vi "InternalStructPos.vi"() -> ()   [LabVIEW 2015]
uses:
  GlobalPath.vi
  GlobalData.vi
  GlobalVi.vi
panel:
  in  "ptfe 9":bool caption="Position the 2 cooling bars"
  in  "Done?":bool
  in  "ptfe 6":bool caption="Connect the mass ground jumpers among the 6 external frames"
  in  "ptfe 5":bool caption="Screw the 20 mass grounds to the frames (internal+external)"
  in  "ptfe 4":bool caption="Position the 5 honeycomb sheets"
  in  "ptfe 3":bool caption="Position the 4 internal frames"
  in  "ptfe 2":bool caption="Position the 6 external frames using 12 PTFE pins"
  # "Internal Structure Positioning"
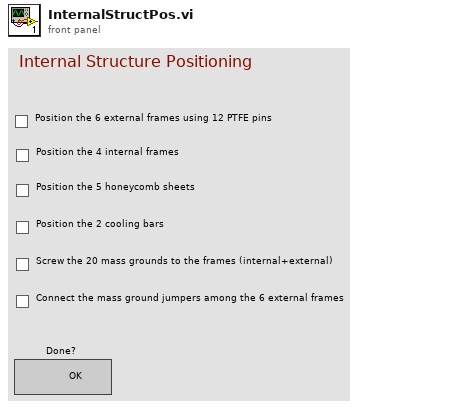
[diagram p1: front panel]
types:
  T1 = enum16{"open", "replace", "create", "open or create", "replace or create", "replace or create with confirmation"}
  T2 = enum32{"Bad", "Idle", "Run top level", "Running"}
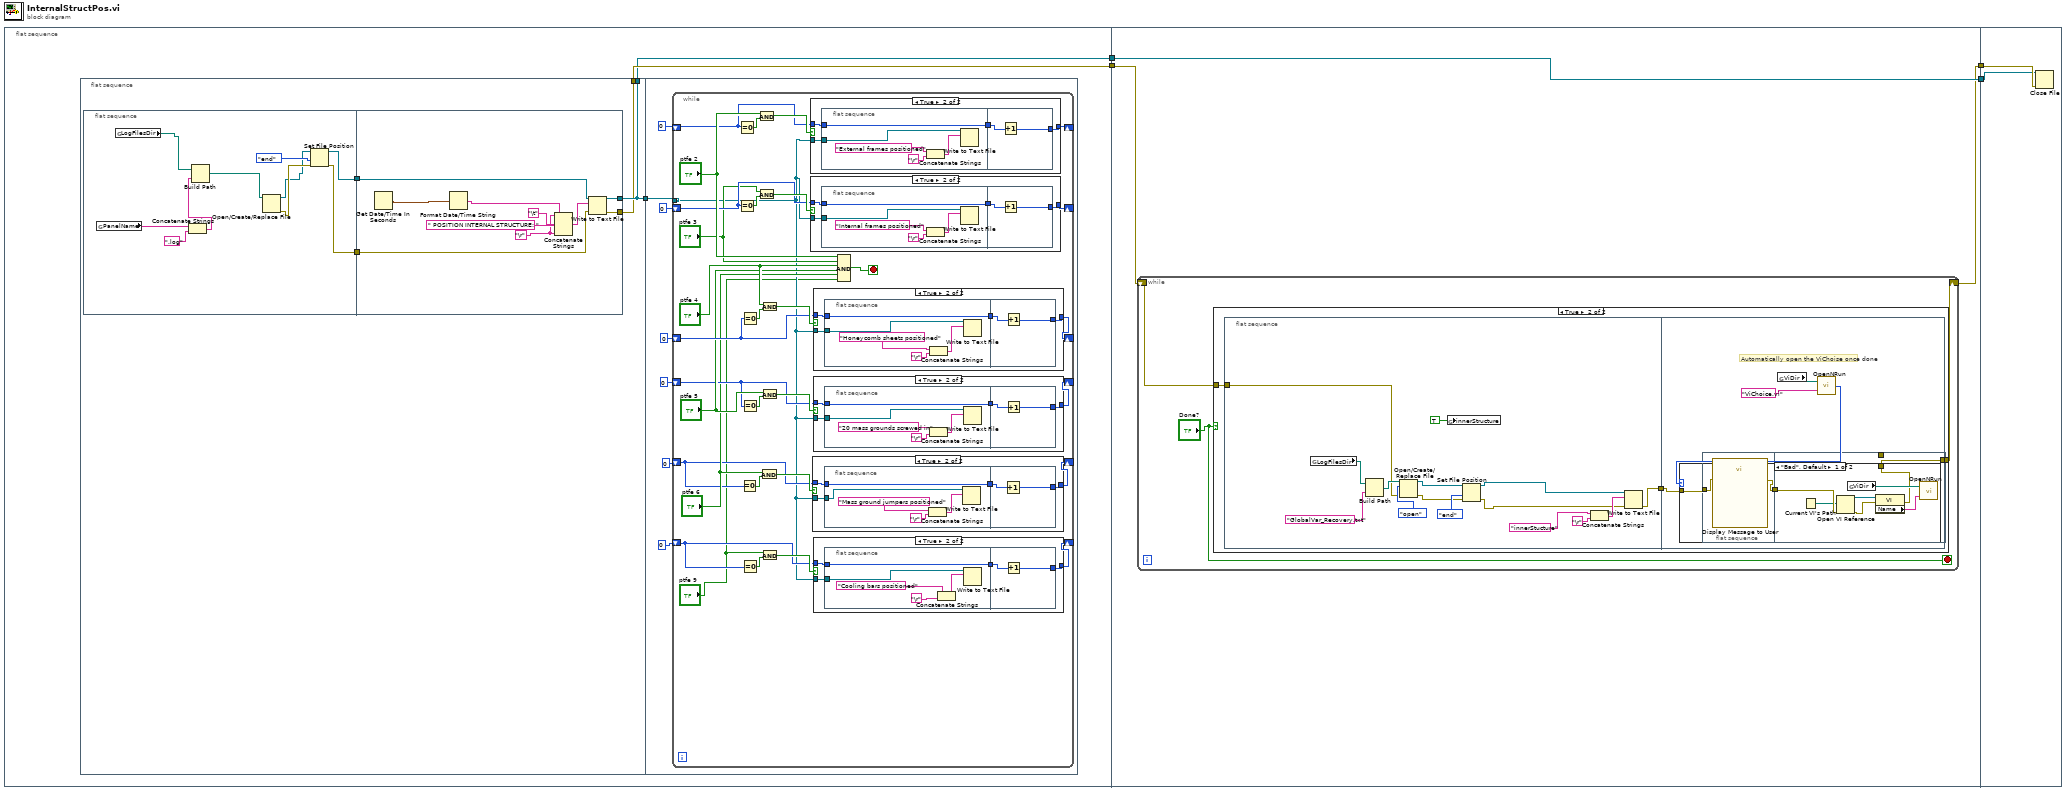
[diagram p0: block diagram]
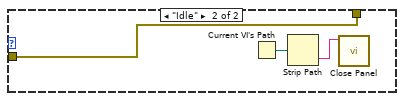
[diagram p9: hidden frame]
diagram:
  n1 = flat-sequence {
    tunnel: [w6] -> w3
    tunnel: [w5] -> w2
    tunnel: [w144] -> w4
    tunnel: w3 -> [w143]
    tunnel: w2 -> [w145]
    tunnel: [w145] -> w1
    tunnel: w4 -> [w189]
    tunnel: w1 -> [w188]
    frame #0 {
      n2 = flat-sequence {
        tunnel: [w10] -> w7
        tunnel: [w10] -> w5
        tunnel: [w9] -> w6
        tunnel: w7 -> [w38]
        frame #0 {
          n3 = flat-sequence {
            tunnel: [w13] -> w11
            tunnel: [w15] -> w8
            tunnel: w11 -> [w27]
            tunnel: [w26] -> w10
            tunnel: [w25] -> w9
            tunnel: w8 -> [w24]
            frame #0 {
              n4 = global read "GlobalData.vi" "PanelName"() -> (w20:string)
              n5 = global read "GlobalPath.vi" "LogFilesDir"() -> (w12:path)
              n6 = Concatenate Strings(w20, ".log") -> (w19:string)
              n7 = Build Path(base path=w12, name or relative path=w19) -> (appended path=w18:path)
              n8 = Open/Create/Replace File(file path (use dialog)=w18) -> (refnum out=w14:refnum<file>, error out=w16:errorcluster)  [unwired: 5 in, 1 out]
              n9 = Set File Position(refnum=w14, from (0:start)=enum16{"start", "end", "current"}."end", error in=w16) -> (refnum out=w13:refnum<file>, error out=w15:errorcluster)  [unwired: 1 in]
            }
            frame #1 {
              w22 = "\r"
              n10 = Get Date/Time In Seconds() -> (seconds since 1Jan1904=w23:timestamp)
              n11 = Format Date/Time String(seconds (now)=w23) -> (date/time string=w29:string)  [unwired: 2 in]
              n12 = Concatenate Strings(w22, w29, "\t", " POSITION INTERNAL STRUCTURE: ", w22) -> (w28:string)
              n13 = Write to Text File(file (use dialog)=w27, text=w28, error in=w24) -> (refnum out=w26:refnum<file>, error out=w25:errorcluster)  [unwired: 1 in, 1 out]
            }
          }
        }
        frame #1 {
          n14 = while {
            tunnel: w38 -> [w40]
            shift-right: [w65] -> _
            shift-left: 0 -> [w66]
            shift-right: [w61] -> _
            shift-left: 0 -> [w62]
            shift-right: [w55] -> _
            shift-left: 0 -> [w57]
            shift-right: [w50] -> _
            shift-left: 0 -> [w51]
            shift-right: [w45] -> _
            shift-left: 0 -> [w46]
            shift-right: [w41] -> _
            shift-left: 0 -> [w42]
            stop <- w70 stop-if-true
            n15 = Equal To 0?(x=w66) -> (x = 0?=w69:bool)
            n16 = Equal To 0?(x=w62) -> (x = 0?=w64:bool)
            n17 = Equal To 0?(x=w46) -> (x = 0?=w49:bool)
            n18 = Equal To 0?(x=w57) -> (x = 0?=w59:bool)
            n19 = Equal To 0?(x=w51) -> (x = 0?=w54:bool)
            n20 = Equal To 0?(x=w42) -> (x = 0?=w44:bool)
            n21 = And(x="ptfe 2", y=w69) -> (x .and. y?=w68:bool)
            n22 = And(x="ptfe 3", y=w64) -> (x .and. y?=w63:bool)
            n23 = And(x="ptfe 6", y=w49) -> (x .and. y?=w48:bool)
            n24 = And(x="ptfe 4", y=w59) -> (x .and. y?=w58:bool)
            n25 = And(x="ptfe 5", y=w54) -> (x .and. y?=w53:bool)
            n26 = And(x="ptfe 9", y=w44) -> (x .and. y?=w43:bool)
            n27 = case shown="True" w68 {
              tunnel: w40 -> [_ w135]
              tunnel: w66 -> [w131 w133]
              tunnel: [w131 w132] -> w65
              frame False {
              }
              frame True {
                n28 = flat-sequence {
                  tunnel: w135 -> [w138]
                  tunnel: [w137] -> w134
                  tunnel: w133 -> [w137]
                  tunnel: w134 -> [w142]
                  tunnel: [w141] -> w132
                  frame #0 {
                    n29 = Concatenate Strings("External frames positioned", "\r") -> (w140:string)
                    n30 = Write to Text File(file (use dialog)=w138, text=w140) -> ()  [unwired: 2 in, 3 out]
                  }
                  frame #1 {
                    n31 = Increment(x=w142) -> (x+1=w141:i32)
                  }
                }
              }
            }
            n32 = case shown="True" w63 {
              tunnel: w40 -> [_ w123]
              tunnel: w62 -> [w119 w121]
              tunnel: [w119 w120] -> w61
              frame False {
              }
              frame True {
                n33 = flat-sequence {
                  tunnel: w123 -> [w126]
                  tunnel: [w125] -> w122
                  tunnel: w121 -> [w125]
                  tunnel: w122 -> [w130]
                  tunnel: [w129] -> w120
                  frame #0 {
                    n34 = Concatenate Strings("Internal frames positioned", "\r") -> (w128:string)
                    n35 = Write to Text File(file (use dialog)=w126, text=w128) -> ()  [unwired: 2 in, 3 out]
                  }
                  frame #1 {
                    n36 = Increment(x=w130) -> (x+1=w129:i32)
                  }
                }
              }
            }
            n37 = case shown="True" w48 {
              tunnel: w40 -> [_ w87]
              tunnel: w46 -> [w83 w85]
              tunnel: [w83 w84] -> w45
              frame False {
              }
              frame True {
                n38 = flat-sequence {
                  tunnel: w87 -> [w90]
                  tunnel: [w89] -> w86
                  tunnel: w85 -> [w89]
                  tunnel: w86 -> [w94]
                  tunnel: [w93] -> w84
                  frame #0 {
                    n39 = Concatenate Strings("Mass ground jumpers positioned", "\r") -> (w92:string)
                    n40 = Write to Text File(file (use dialog)=w90, text=w92) -> ()  [unwired: 2 in, 3 out]
                  }
                  frame #1 {
                    n41 = Increment(x=w94) -> (x+1=w93:i32)
                  }
                }
              }
            }
            n42 = case shown="True" w58 {
              tunnel: w40 -> [_ w111]
              tunnel: w57 -> [w107 w109]
              tunnel: [w107 w108] -> w55
              frame False {
              }
              frame True {
                n43 = flat-sequence {
                  tunnel: w111 -> [w114]
                  tunnel: [w113] -> w110
                  tunnel: w109 -> [w113]
                  tunnel: w110 -> [w118]
                  tunnel: [w117] -> w108
                  frame #0 {
                    n44 = Concatenate Strings("Honeycomb sheets positioned", "\r") -> (w116:string)
                    n45 = Write to Text File(file (use dialog)=w114, text=w116) -> ()  [unwired: 2 in, 3 out]
                  }
                  frame #1 {
                    n46 = Increment(x=w118) -> (x+1=w117:i32)
                  }
                }
              }
            }
            n47 = case shown="True" w53 {
              tunnel: w40 -> [_ w99]
              tunnel: w51 -> [w95 w97]
              tunnel: [w95 w96] -> w50
              frame False {
              }
              frame True {
                n48 = flat-sequence {
                  tunnel: w99 -> [w102]
                  tunnel: [w101] -> w98
                  tunnel: w97 -> [w101]
                  tunnel: w98 -> [w106]
                  tunnel: [w105] -> w96
                  frame #0 {
                    n49 = Concatenate Strings("20 mass grounds screwed in", "\r") -> (w104:string)
                    n50 = Write to Text File(file (use dialog)=w102, text=w104) -> ()  [unwired: 2 in, 3 out]
                  }
                  frame #1 {
                    n51 = Increment(x=w106) -> (x+1=w105:i32)
                  }
                }
              }
            }
            n52 = case shown="True" w43 {
              tunnel: w40 -> [_ w75]
              tunnel: w42 -> [w71 w73]
              tunnel: [w71 w72] -> w41
              frame False {
              }
              frame True {
                n53 = flat-sequence {
                  tunnel: w75 -> [w78]
                  tunnel: [w77] -> w74
                  tunnel: w73 -> [w77]
                  tunnel: w74 -> [w82]
                  tunnel: [w81] -> w72
                  frame #0 {
                    n54 = Concatenate Strings("Cooling bars positioned", "\r") -> (w80:string)
                    n55 = Write to Text File(file (use dialog)=w78, text=w80) -> ()  [unwired: 2 in, 3 out]
                  }
                  frame #1 {
                    n56 = Increment(x=w82) -> (x+1=w81:i32)
                  }
                }
              }
            }
            n57 = Compound Arithmetic op=AND("ptfe 2", "ptfe 3", "ptfe 4", "ptfe 5", "ptfe 6", "ptfe 9") -> (w70:bool)
          }
        }
      }
    }
    frame #1 {
      n58 = while {
        shift-right: [w148] -> w144
        shift-left: w143 -> [w147]
        stop <- "Done?" stop-if-true
        n59 = case shown="True" "Done?" {
          tunnel: [w149 w152] -> w148
          tunnel: w147 -> [w149 w151]
          frame False {
          }
          frame True {
            n60 = flat-sequence {
              tunnel: w151 -> [w156]
              tunnel: [w155] -> w150
              tunnel: [w169] -> w152
              tunnel: w150 -> [w168]
              frame #0 {
                n61 = global read "GlobalPath.vi" "LogFilesDir"() -> (w153:path)
                n62 = Build Path(base path=w153, name or relative path="GlobalVar_Recovery.txt") -> (appended path=w165:path)
                n63 = Open/Create/Replace File(file path (use dialog)=w165, error in=w156, operation (0:open)=T1."open") -> (refnum out=w161:refnum<file>, error out=w162:errorcluster)  [unwired: 3 in, 1 out]
                n64 = global write "GlobalVi.vi" "innerStructure"(TRUE) -> ()
                n65 = Set File Position(refnum=w161, from (0:start)=enum16{"start", "end", "current"}."end", error in=w162) -> (refnum out=w158:refnum<file>, error out=w157:errorcluster)  [unwired: 1 in]
                n66 = Concatenate Strings("innerStucture", "\r") -> (w160:string)
                n67 = Write to Text File(file (use dialog)=w158, text=w160, error in=w157) -> (error out=w155:errorcluster)  [unwired: 1 in, 2 out]
              }
              frame #1 {
                # "Automatically open the ViChoise once done"
                n68 = global read "GlobalPath.vi" "ViDir"() -> (w172:path)
                n69 = call "OpenNRun.vi"("VI name"="ViChoice.vi", "ViDirPath"=w172) -> ("Execution:State"=w171:T2)
                n70 = case shown="\"Bad\", Default" w171 {
                  tunnel: [w173 w185] -> w169
                  tunnel: w168 -> [w174 w185]
                  frame "Bad", Default {
                    n71 = flat-sequence {
                      tunnel: w174 -> [w177]
                      tunnel: [w176] -> w175
                      tunnel: w175 -> [w181]
                      tunnel: [w178] -> w173
                      frame #0 {
                        n72 = call "Display Message to User"("error in (no error)"=w177) -> ("error out"=w176:errorcluster)  [unwired: 9 in, 1 out]
                      }
                      frame #1 {
                        n73 = Current VI's Path() -> (path=w179:path)
                        n74 = Open VI Reference(vi path=w179, error in (no error)=w181) -> (vi reference=w184:refnum<vi>, error out=w183:errorcluster)  [unwired: 4 in]
                        n75 = global read "GlobalPath.vi" "ViDir"() -> (w180:path)
                        n76 = property class="VI"(reference=w184, error in=w183) -> (error out=w178:errorcluster, "Name"=w182:string)  [unwired: 1 out]
                        n77 = call "OpenNRun.vi"("VI name"=w182, "ViDirPath"=w180) -> ()  [unwired: 1 out]
                      }
                    }
                  }
                  frame "Idle" {
                    n78 = Current VI's Path() -> (path=w186:path)
                    n79 = Strip Path(path=w186) -> (name=w187:string)  [unwired: 1 out]
                    n80 = call <vilib>:"Close Panel.vi"("VI name"=w187) -> ()  [unwired: 10 in, 1 out]
                  }
                }
              }
            }
          }
        }
      }
    }
    frame #2 {
      n81 = Close File(refnum=w188, error in=w189) -> ()  [unwired: 2 out]
    }
  }
